vi "Fibonacci LFSRs -pseudo random.vi"(11 "reset random":bool) -> (3 "rand number":u16)   [LabVIEW 2021]
doc: "genarate pasodo random number.\nhttps://en.wikipedia.org/wiki/Linear-feedback_shift_register"
panel:
  # "tested, its has a flat histogram!"
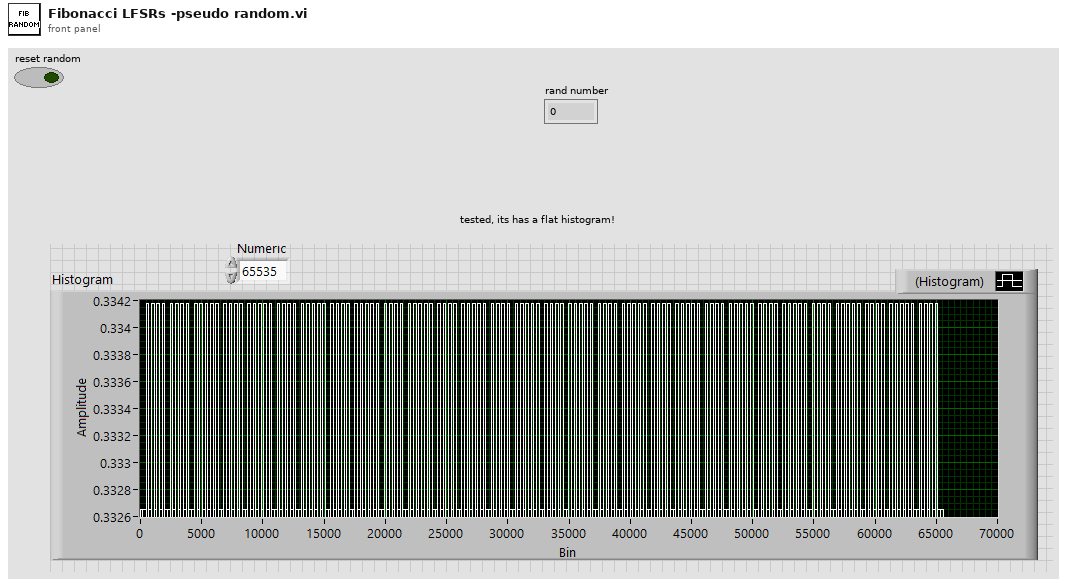
[diagram p1: front panel]
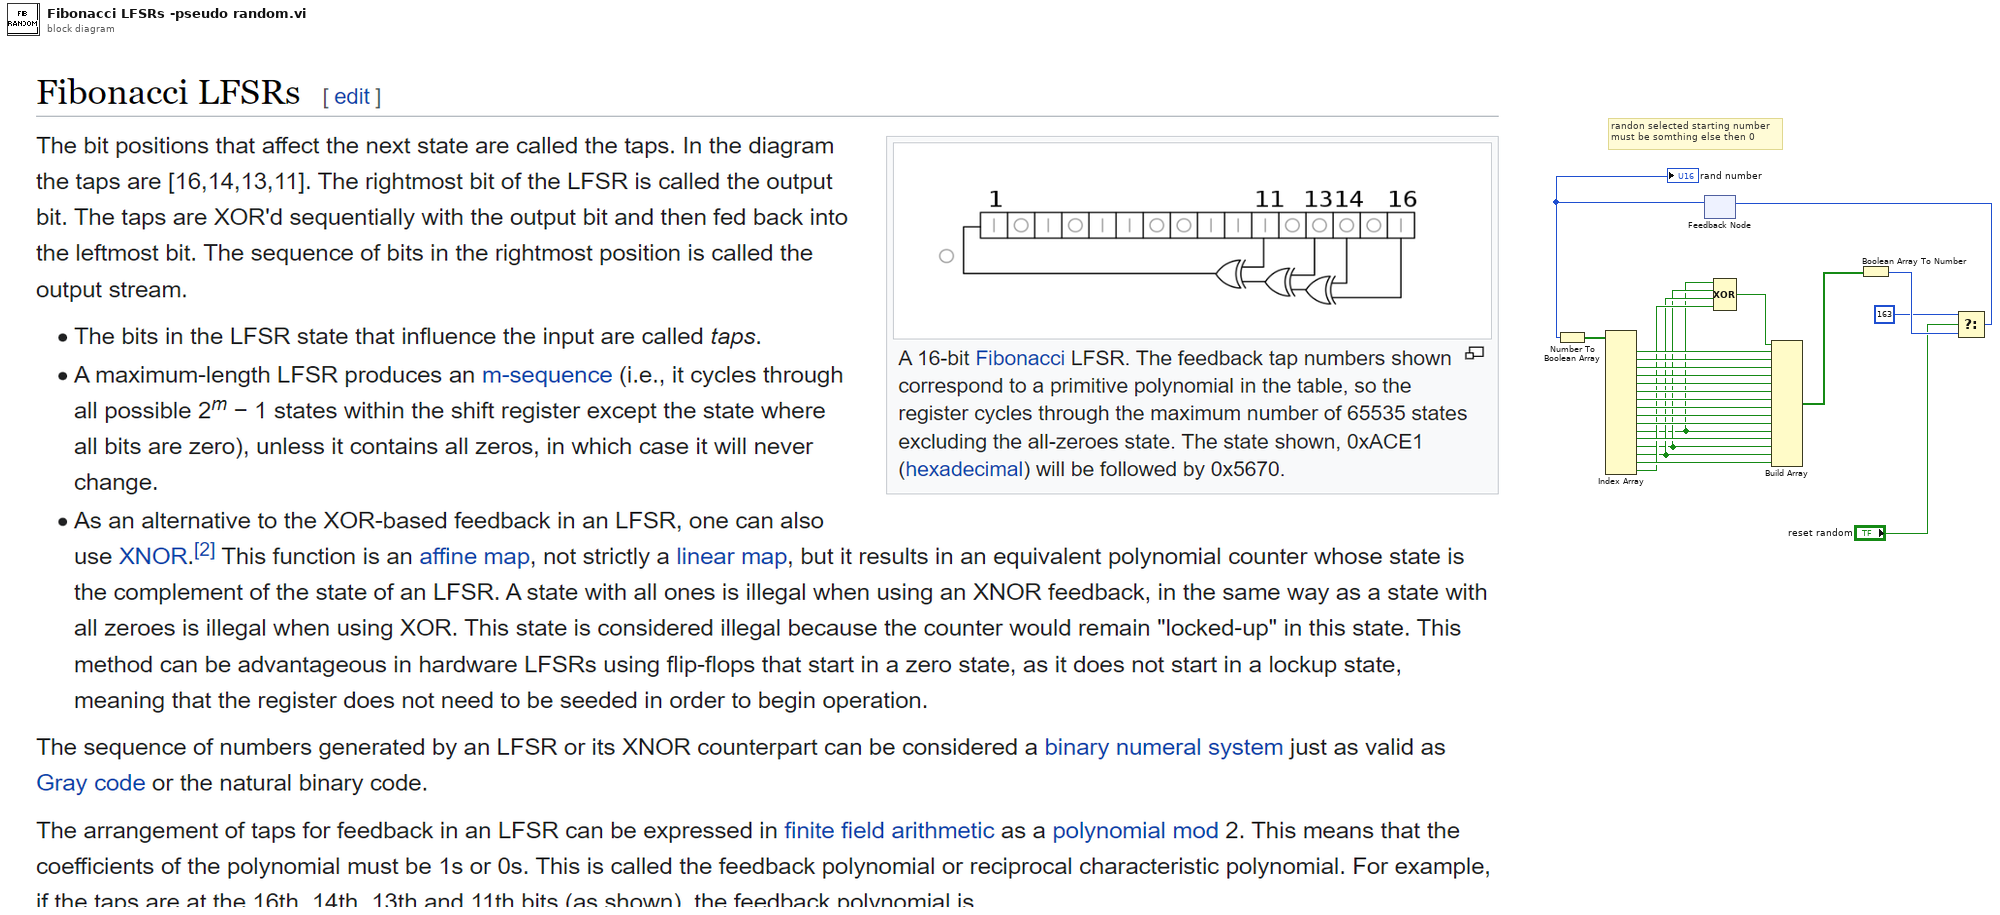
[diagram p0: block diagram]
diagram:
  # "randon selected starting number\nmust be somthing else then 0"
  n1 = feedback #1() -> (w5:u16)  [unwired: 1 in]
  "rand number" <- w5
  n2 = Number To Boolean Array(number=w5) -> (Boolean array=w24:bool[])
  n3 = Index Array(array=w24) -> (element #1=w22:bool, element #2=w21:bool, element #3=w20:bool, element #4=w19:bool, element #5=w18:bool, element #6=w17:bool, element #7=w16:bool, element #8=w15:bool, element #9=w14:bool, element #10=w13:bool, element #11=w7:bool, element #12=w12:bool, element #13=w8:bool, element #14=w9:bool, element #15=w11:bool, element #16=w10:bool)  [unwired: 16 in]
  n4 = Compound Arithmetic op=XOR(w7, w8, w9, w10) -> (w23:bool)
  n5 = Build Array(w23, w22, w21, w20, w19, w18, w17, w16, w15, w14, w13, w7, w12, w8, w9, w11) -> (w6:bool[])
  n6 = Boolean Array To Number(Boolean array=w6) -> (number=w4:u16)
  n7 = Select(t=u16 163, s="reset random", f=w4) -> (s? t:f=w1:u16)
  n8 = feedback-in #1(w1) -> ()
